vi "GetResolution.vi"(8 "error in (no error)":errorcluster, 11 "CameraDemo in":refnum<class "Camera.lvclass">) -> (0 "error out":errorcluster, 2 "Resolution":u8 format="%.0x", 3 "CameraDemo out":refnum<class "Camera.lvclass">)   [LabVIEW 2020, in "CameraI2COUSB.lvlib" / "Camera.lvclass"]
uses:
  Camera.lvclass
  Camera.lvclass/Camera.ctl
  Private/TypeDef/RegisterName.ctl
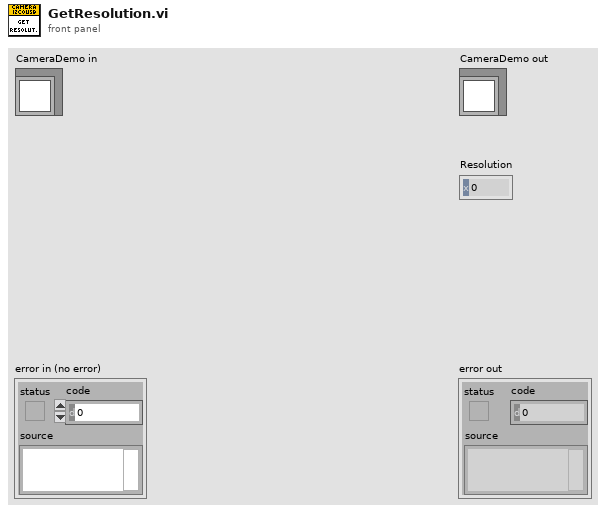
[diagram p1: front panel]
types:
  T1 = typedef "CameraI2COUSB.lvlib/Camera.lvclass/RegisterName.ctl" = enum16{"Clock Rate", "Frame Rate", "Image Type", "Resolution", "Snap", "Start Streaming", "Stop Streaming"}
  T2 = typedef "CameraI2COUSB.lvlib/Camera.lvclass/RegisterInfo.ctl" = cluster{"Address":u16, "Lenght":u32}
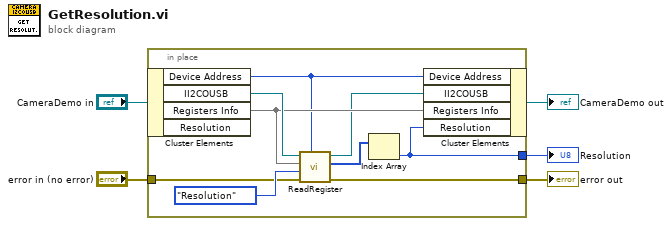
[diagram p0: block diagram]
diagram:
  n1 = in-place {
    in-place-border: "error in (no error)" -> [w10]
    in-place-border: [w9] -> w1
    in-place-border: [w8] -> w5
    n2 = in-place-cluster #1("CameraDemo in") -> ("Device Address"=w11:u8, "II2COUSB"=w14:refnum<class "II2COUSB.lvclass">, "Registers Info"=w13:map{T1, T2})  [unwired: 1 out]
    n3 = call "ReadRegister.vi"("Device Address"=w11, "error in (no error)"=w10, "Register Name"=RegisterName."Resolution", "Registers Info"=w13, "II2COUSB"=w14) -> ("error out"=w9:errorcluster, "DATA"=w7:u8[], "II2COUSB out"=w6:refnum<class "II2COUSB.lvclass">)  [unwired: 4 in]
    n4 = Index Array(array=w7) -> (element=w8:u8)  [unwired: 1 in]
    n5 = in-place-cluster #1("Device Address"=w11, "II2COUSB"=w6, "Registers Info"=w13, "Resolution"=w8) -> (→"CameraDemo out":refnum<class "Camera.lvclass">)
  }
  "error out" <- w1
  "Resolution" <- w5
